vi "Read Config.vi"(11 "Refnum in":T2) -> (1 "local":T1, 2 "server":T1)   [LabVIEW 2017]
uses:
  <vilib>/Utility/config.llb/Config Data RefNum.ctl
  <vilib>/Utility/config.llb/Read Key (String).vi
  <vilib>/Utility/config.llb/NI_LVConfig.lvlib
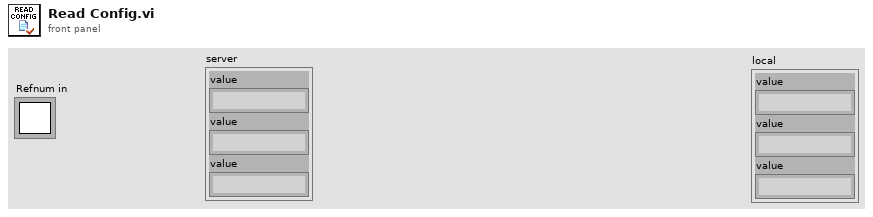
[diagram p1: front panel]
types:
  T1 = cluster{"value":string, "value":string, "value":string}
  T2 = typedef "NI_LVConfig.lvlib/Config Data RefNum.ctl" = refnum<k1>
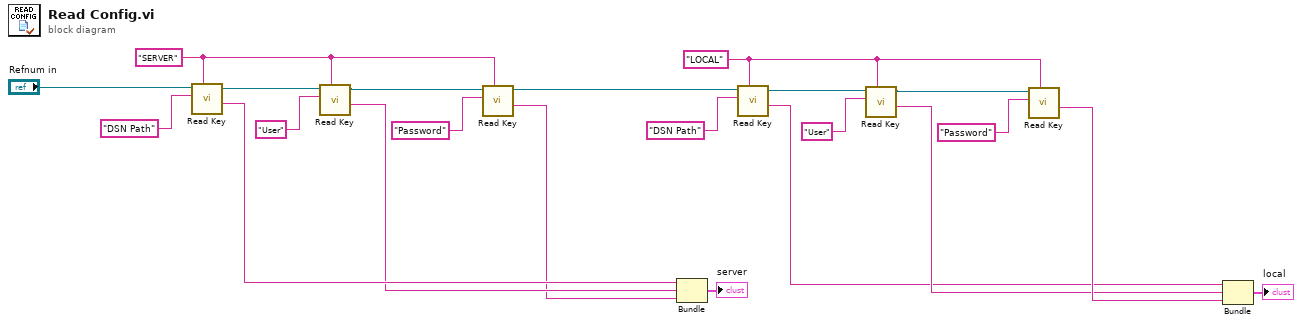
[diagram p0: block diagram]
diagram:
  w2 = "LOCAL" ("section")
  w22 = "SERVER" ("section")
  n1 = call-poly <vilib>:"Read Key.vi"("section"=w22, "key"="DSN Path", "refnum"="Refnum in") -> ("value"=w15:string, "refnum out"=w19:T2)  [unwired: 5 in, 2 out]
  n2 = call-poly <vilib>:"Read Key.vi"("section"=w22, "key"="User", "refnum"=w19) -> ("value"=w14:string, "refnum out"=w21:T2)  [unwired: 5 in, 2 out]
  n3 = call-poly <vilib>:"Read Key.vi"("section"=w22, "key"="Password", "refnum"=w21) -> ("value"=w13:string, "refnum out"=w1:T2)  [unwired: 5 in, 2 out]
  n4 = Bundle("value"=w15, "value"=w14, "value"=w13) -> (→"server":T1)  [unwired: 1 in]
  n5 = call-poly <vilib>:"Read Key.vi"("section"=w2, "key"="DSN Path", "refnum"=w1) -> ("value"=w8:string, "refnum out"=w5:T2)  [unwired: 5 in, 2 out]
  n6 = call-poly <vilib>:"Read Key.vi"("section"=w2, "key"="User", "refnum"=w5) -> ("value"=w9:string, "refnum out"=w3:T2)  [unwired: 5 in, 2 out]
  n7 = call-poly <vilib>:"Read Key.vi"("section"=w2, "key"="Password", "refnum"=w3) -> ("value"=w10:string)  [unwired: 5 in, 3 out]
  n8 = Bundle("value"=w8, "value"=w9, "value"=w10) -> (→"local":T1)  [unwired: 1 in]
